vi "Configure Offsets.vi"(7 "Config Folder":path, 8 "error in (no error)":errorcluster, 11 "WorkTable Class in":refnum<class "WorkTable Class.lvclass">) -> (0 "error out":errorcluster, 3 "WorkTable Class out":refnum<class "WorkTable Class.lvclass">)   [LabVIEW 2011, in "WorkTable Class.lvclass"]
uses:
  WorkTable Class.lvclass
  WorkTable Class.lvclass/WorkTable Class.ctl
  <vilib>/Utility/config.llb/Read Key (String).vi
  <vilib>/Utility/config.llb/NI_LVConfig.lvlib
  Vec3d Class/Vec3d Class.lvclass
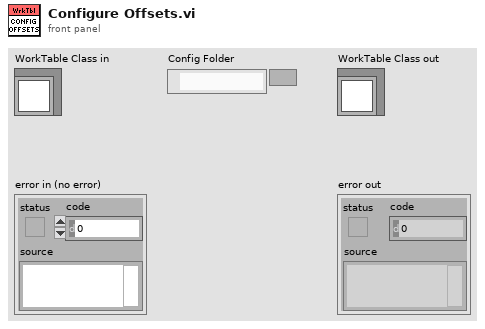
[diagram p1: front panel]
types:
  T1 = typedef "NI_LVConfig.lvlib/Config Data RefNum.ctl" = refnum<k1>
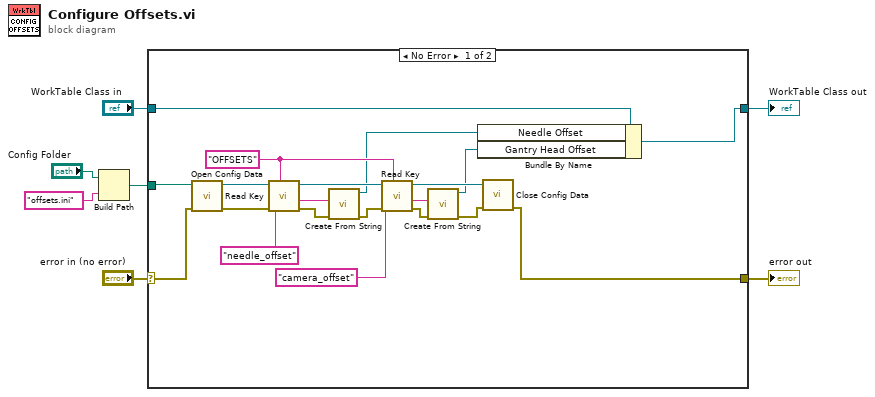
[diagram p0: block diagram]
diagram:
  n1 = Build Path(base path="Config Folder", name or relative path="offsets.ini") -> (appended path=w1:path)
  n2 = case shown="No Error" "error in (no error)" {
    selector: "error in (no error)" -> [w9 w29]
    tunnel: [w8 w29] -> w6
    tunnel: [w12 w28] -> w4
    tunnel: "WorkTable Class in" -> [w13 w28]
    tunnel: w1 -> [w27 _]
    frame No Error {
      w18 = "OFFSETS" ("section")
      n3 = call <vilib>:"Open Config Data.vi"("error in (no error)"=w9, "configuration file path"=w27) -> ("error out"=w22:errorcluster, "refnum"=w26:T1)  [unwired: 7 in, 1 out]
      n4 = call-poly <vilib>:"Read Key.vi"("section"=w18, "error in (no error)"=w22, "key"="needle_offset", "refnum"=w26) -> ("error out"=w23:errorcluster, "value"=w24:string, "refnum out"=w21:T1)  [unwired: 4 in, 1 out]
      n5 = call "Create From String.vi"("error in"=w23, "Input String"=w24) -> ("error out"=w20:errorcluster, "Vec3d out"=w11:refnum<class "Vec3d Class.lvclass">)  [unwired: 8 in]
      n6 = call-poly <vilib>:"Read Key.vi"("section"=w18, "error in (no error)"=w20, "key"="camera_offset", "refnum"=w21) -> ("error out"=w16:errorcluster, "value"=w17:string, "refnum out"=w15:T1)  [unwired: 4 in, 1 out]
      n7 = call "Create From String.vi"("error in"=w16, "Input String"=w17) -> ("error out"=w14:errorcluster, "Vec3d out"=w10:refnum<class "Vec3d Class.lvclass">)  [unwired: 8 in]
      n8 = Bundle By Name(cluster=w13, "Needle Offset"=w11, "Gantry Head Offset"=w10) -> (w12:refnum<class "WorkTable Class.lvclass">)
      n9 = call <vilib>:"Close Config Data.vi"("error in (no error)"=w14, "refnum"=w15) -> ("error out"=w8:errorcluster)  [unwired: 8 in, 1 out]
    }
    frame Error {
    }
  }
  "error out" <- w6
  "WorkTable Class out" <- w4
